vi "Dice.vi"() -> ()   [LabVIEW 2017]
panel:
  in  "stop":bool
  in  "OK Button":bool
  out "Pict Ring":u8(ring)
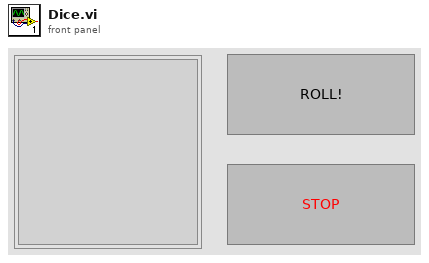
[diagram p1: front panel]
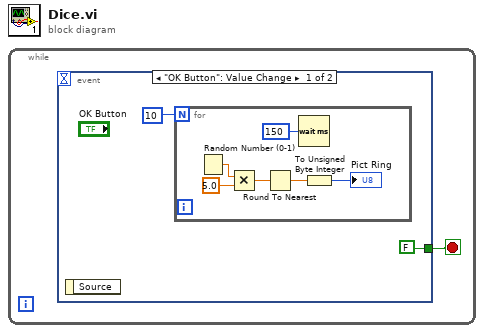
[diagram p0: block diagram]
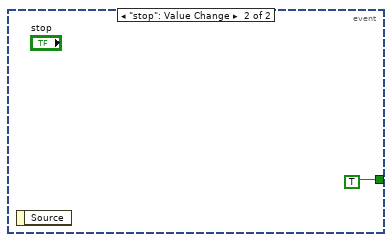
[diagram p2: hidden frame]
diagram:
  n1 = while {
    stop <- w1 stop-if-true
    n2 = event shown="[0] \"OK Button\": Value Change" {
      selector: _ -> [_ _]
      dyn-events: _ -> [_ _]
      timeout: _ -> [_ _]
      tunnel: [FALSE TRUE] -> w1
      event "OK Button": Value Change {
        n3 = event-data() -> ()  [unwired: 1 in, 1 out]
        n4 = for {
          N: 10 ("Numeric Control") -> [_]
          n5 = Random Number (0-1)() -> (number: 0 to 1=w9:dbl)
          n6 = Multiply(x=w9, y=5.0) -> (x*y=w7:dbl)
          n7 = Round To Nearest(number=w7) -> (nearest integer value=w6:dbl)
          n8 = Wait (ms)(milliseconds to wait=u32 150) -> ()  [unwired: 1 out]
          n9 = To Unsigned Byte Integer(number=w6) -> (unsigned 8bit integer=→"Pict Ring":u8)
        }
      }
      event "stop": Value Change {
        n10 = event-data() -> ()  [unwired: 1 in, 1 out]
      }
    }
  }
